vi "DisplayGeneralConfig.vi"(11 "Cluster in":refnum<vi>) -> ()   [LabVIEW 2014]
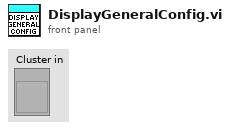
[diagram p1: front panel]
types:
  T1 = cluster{"PCM_CAN_ID":dbl, "PDP_CAN_ID":dbl, "PodCount":dbl, "BaseRobotMass":dbl, "Caution":string}
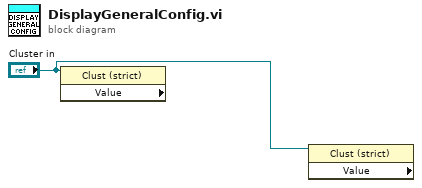
[diagram p0: block diagram]
diagram:
  n1 = property class="Clust (strict)"(reference="Cluster in") -> ("Value"=w2:T1)  [unwired: 1 in, 2 out]
  n2 = property class="Clust (strict)"(reference="Cluster in") -> ("Value"=w3:T1)  [unwired: 1 in, 2 out]
